vi "Read_Coils_Output.vi"() -> ()   [LabVIEW 2016]
uses:
  <vilib>/NI/Current Value Table/DataTypes/Boolean_Read.vi
  <vilib>/NI/Current Value Table/Type to Enum.vi
  <vilib>/NI/Current Value Table/DataTypes/Boolean_Type To Enum.vi
  <vilib>/Utility/file.llb/Read Delimited Spreadsheet (string).vi
  <vilib>/NI/Current Value Table/FGVs/CVT Globals.vi
  <vilib>/NI/Current Value Table/FGVs/Tag Memory.vi
  <vilib>/NI/Current Value Table/Memory Block.vi
  <vilib>/NI/Current Value Table/DataTypes/Boolean_Memory Block.vi
  <vilib>/NI/Current Value Table/Current Value Table.lvlib
panel:
  out "subarray 3":cluster{bool}[](array[cluster])
  out "subarray":cluster{bool}[](array[cluster])
  in  "Back to Main Page":bool
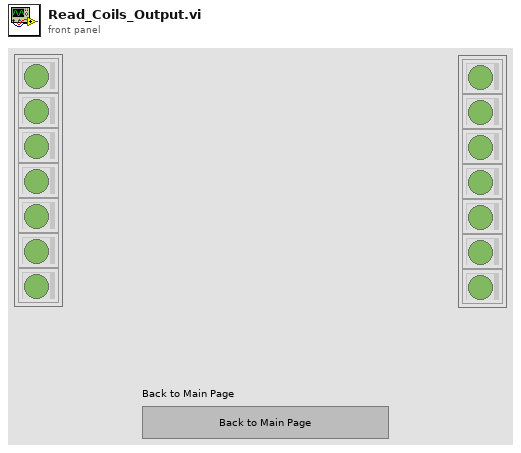
[diagram p1: front panel]
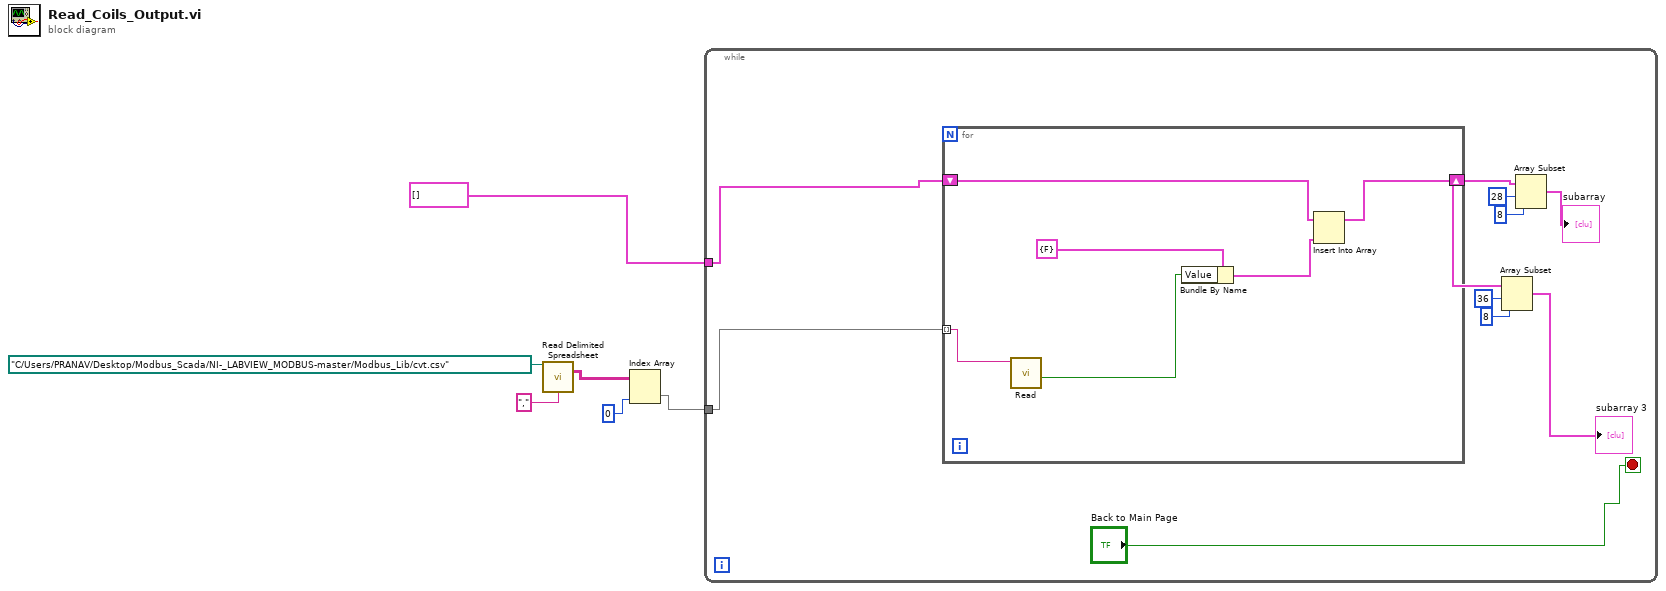
[diagram p0: block diagram]
diagram:
  n1 = call-poly <vilib>:"Read Delimited Spreadsheet.vi"("file path (dialog if empty)"=path "C:/Users/PRANAV/Desktop/Modbus_Scada/NI-_LABVIEW_MODBUS-master/Modbus_Lib/cvt.csv", "delimiter (\\t)"="," ("delimiter (\\t)")) -> ("all rows"=w2:string[][])  [unwired: 8 in, 5 out]
  n2 = Index Array "Index Array"(array=w2, index (col)=0 ("disabled index (col)")) -> (element=w4:string[])  [unwired: 1 in]
  n3 = while {
    tunnel: cluster{"Value":bool}[] [] ("output array") -> [w9]
    tunnel: w4 -> [w8]
    stop <- "Back to Main Page" stop-if-true
    n4 = for {
      shift-right: [w17] -> w15
      shift-left: w9 -> [w21]
      tunnel: w8 -> [w22] mode=indexing
      n5 = call-poly <vilib>:"Read.vi"("Tag Name"=w22) -> ("Value"=w19:bool)  [unwired: 9 in, 1 out]
      n6 = Bundle By Name(cluster=cluster{"Value":bool} {"Value"=FALSE} ("Cluster"), "Value"=w19) -> (w18:cluster{"Value":bool})
      n7 = Insert Into Array "Insert Into Array"(array=w21, new element=w18) -> (w17:cluster{"Value":bool}[])  [unwired: 1 in]
    }
    n8 = Array Subset(array=w15, index=36, length=8) -> (→"subarray 3":cluster{"Value":bool}[])
    n9 = Array Subset(array=w15, index=28, length=8) -> (→"subarray":cluster{"Value":bool}[])
  }
